vi "Destroy Monitor Log (pcap).vi"(8 "error in":errorcluster, 10 "pcap_dumper_t":u64, 11 "pcap_t out":u64) -> (0 "error out":errorcluster)   [LabVIEW 2020, in "AIM ARINC 664 Engine.lvlib" / "Implementation.lvlib" / "Monitor Execution Unit.lvclass"]
uses:
  Monitor Execution Unit.lvclass
  libpcaplv/libpcaplv.lvlib
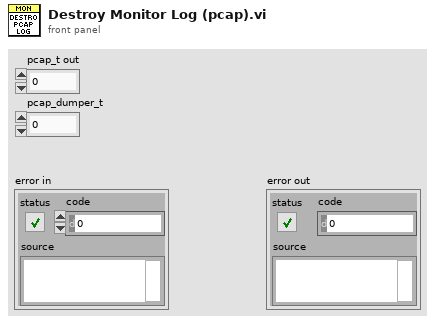
[diagram p1: front panel]
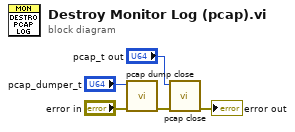
[diagram p0: block diagram]
diagram:
  n1 = call "pcap dump close.vi"("error in"="error in", "pcap_dumper_t in"="pcap_dumper_t") -> ("error out"=w4:errorcluster)  [unwired: 9 in]
  n2 = call "pcap close.vi"("error in"=w4, "pcap_t in"="pcap_t out") -> ("error out"=→"error out":errorcluster)  [unwired: 9 in]
